vi "Exp no 7b Application Using WHILE LOOP.vi"() -> ()   [LabVIEW 2010]
panel:
  out "Sum of Even Numbers":i32
  in  "N":i32
  # "SUM OF EVEN NUMBERS"
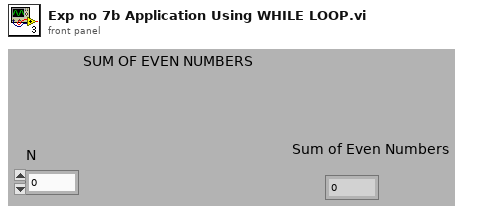
[diagram p1: front panel]
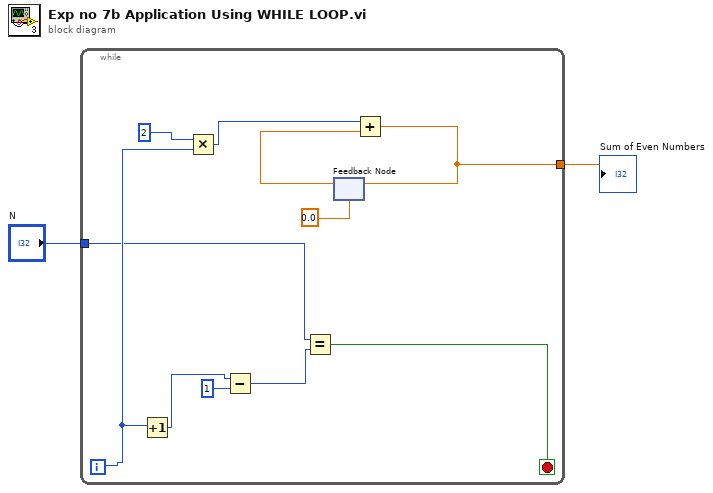
[diagram p0: block diagram]
diagram:
  n1 = while {
    tunnel: "N" -> [w7]
    tunnel: [w3] -> w1
    i -> [w9]
    stop <- w10 stop-if-true
    n2 = Increment(x=w9) -> (x+1=w13:i32)
    n3 = Multiply(x=2, y=w9) -> (x*y=w4:i32)
    n4 = Subtract(x=w13, y=1) -> (x-y=w11:i32)
    n5 = Equal?(x=w7, y=w11) -> (x = y?=w10:bool)
    n6 = feedback #1(0.0) -> (w6:dbl)
    n7 = Add(x=w4, y=w6) -> (x+y=w3:dbl)
    n8 = feedback-in #1(w3) -> ()
  }
  "Sum of Even Numbers" <- w1
